vi "HeidenhainStatusToTermin.vi"(3 "error out 2":errorcluster) -> (14 "concatenated string":string, 17 "error out":errorcluster)   [LabVIEW 2011]
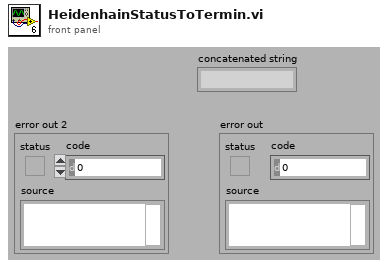
[diagram p1: front panel]
types:
  T1 = cluster{"Fixed Position / [mm] 2":dbl, "Numeric 3":dbl, "Moving Speed / [%] 2":i8, "Differenz 2":dbl, "Actual Microscope Position / [mm] 2":dbl}
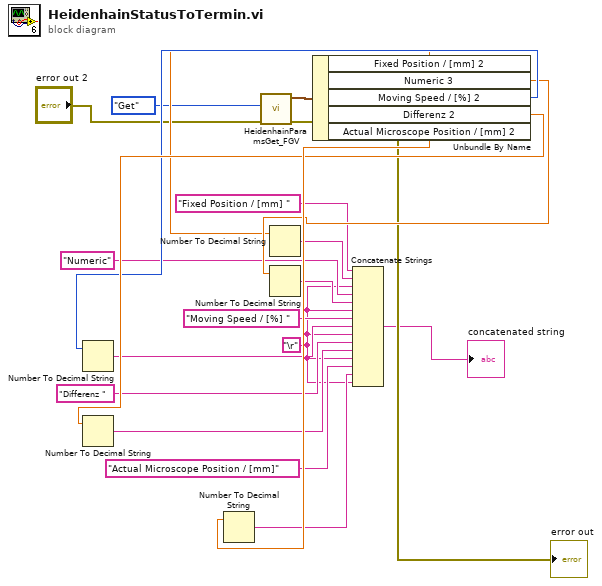
[diagram p0: block diagram]
diagram:
  w1 = "\r"
  n1 = call "HeidenhainParamsGet_FGV.vi"("error in"="error out 2", "FGV_Control"=enum16{"Set", "Get"}."Get") -> ("error out"=→"error out":errorcluster, "out"=w5:T1)  [unwired: 8 in]
  n2 = Unbundle By Name(w5) -> ("Fixed Position / [mm] 2"=w12:dbl, "Numeric 3"=w15:dbl, "Moving Speed / [%] 2"=w17:i8, "Differenz 2"=w18:dbl, "Actual Microscope Position / [mm] 2"=w21:dbl)
  n3 = Number To Decimal String(number=w17) -> (decimal integer string=w16:string)  [unwired: 1 in]
  n4 = Number To Decimal String(number=w18) -> (decimal integer string=w19:string)  [unwired: 1 in]
  n5 = Number To Decimal String(number=w21) -> (decimal integer string=w20:string)  [unwired: 1 in]
  n6 = Number To Decimal String(number=w12) -> (decimal integer string=w13:string)  [unwired: 1 in]
  n7 = Number To Decimal String(number=w15) -> (decimal integer string=w14:string)  [unwired: 1 in]
  n8 = Concatenate Strings("Fixed Position / [mm] " ("string"), w13, w1, "Numeric" ("string"), w14, w1, "Moving Speed / [%] " ("string"), w16, w1, "Differenz " ("string"), w19, w1, "Actual Microscope Position / [mm]" ("string"), w20, w1) -> (→"concatenated string":string)
